vi "LibInit.vi"(8 "error in (no error)":errorcluster) -> (0 "error out":errorcluster)   [LabVIEW 2018, in "LibTiePie.lvlib"]
uses:
  LibTiePie.lvlib
  LabViewHS4/libtiepie.dll
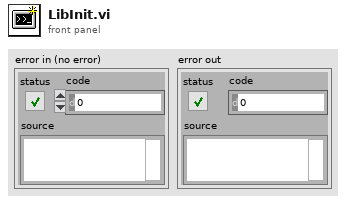
[diagram p1: front panel]
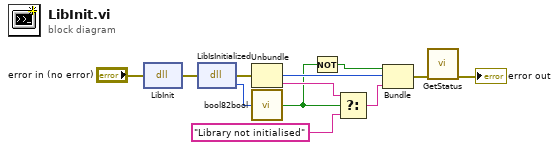
[diagram p0: block diagram]
diagram:
  n1 = dll-call lib="C:/Users/cwaha/Documents/LabViewHS4/libtiepie.dll" fn="LibInit"(error in="error in (no error)") -> (error out=w12:errorcluster)  [unwired: 3 in, 1 out]
  n2 = dll-call lib="C:/Users/cwaha/Documents/LabViewHS4/libtiepie.dll" fn="LibIsInitialized"(error in=w12) -> (error out=w11:errorcluster, "bIsInitialized"=w5:u8)  [unwired: 2 in, 1 out]
  n3 = Unbundle(w11) -> ("code"=w9:i32, "source"=w7:string)  [unwired: 1 out]
  n4 = call "bool82bool.vi"("bool8 in"=w5) -> ("bool out"=w4:bool)
  n5 = Not(x=w4) -> (.not. x?=w3:bool)
  n6 = Select(t=w7, s=w4, f="Library not initialised") -> (s? t:f=w8:string)
  n7 = Bundle(w3, "code"=w9, "source"=w8) -> (w2:cluster{bool, "code":i32, "source":string})  [unwired: 1 in]
  n8 = call "GetStatus.vi"("error in (no error)"=w2) -> ("error out"=→"error out":errorcluster)  [unwired: 10 in]
